vi "VelocidadeDaBolaModulo.vi"(8 "Vy bola":dbl format="%#_13g", 11 "Vx bola":dbl format="%#_13g") -> (3 "Vel bola":dbl format="%#_13g")   [LabVIEW 2017]
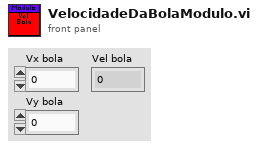
[diagram p1: front panel]
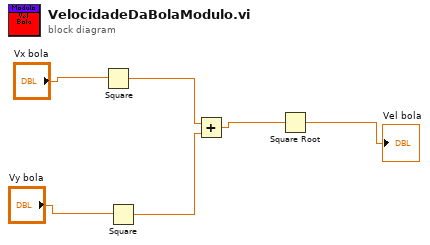
[diagram p0: block diagram]
diagram:
  n1 = Square(x="Vx bola") -> (x^2=w4:dbl)
  n2 = Square(x="Vy bola") -> (x^2=w3:dbl)
  n3 = Add(x=w4, y=w3) -> (x+y=w2:dbl)
  n4 = Square Root(x=w2) -> (sqrt(x)=→"Vel bola":dbl)
